vi "dfd_Create Rational Resampling Filter.vi"(6 "fs":dbl=1.0, 8 "error in (no error)":errorcluster, 10 "rational factor out":T6, 11 "validated numerator":dbl[](array[numeric])) -> (0 "error out":errorcluster, 3 "multirate filter out":T1={"mMRate_Structure"=enum."CIC", "mMRate_Mode"=0, "mMRate_Factor"=0, "mMRate_FIRParams"={"mMRate_FIR_H"=[], "mMRate_FIR_IsNyquist?"=FALSE, "mMRate_FIR_IsSymmetric?"=FALSE}, "mMRate_CICParams"={"mMRate_CIC_#Stage"=0, "mMRate_CIC_Lag"=0, "mMRate_CIC_Type"=enum."Lowpass"}, "mMRate_Order"=0, "mMRate_Version"="", "mMRate_Comments"="", "mMRate_RationalFactor"={"mMRate_L"=-1, "mMRate_M"=-1}, "mMRate_Fs"=0.0, "mMRate_Quantized?"=FALSE, "mMRate_QFilterGain"=1.0, "mMRate_CoefWl"=16, "mMRate_Scaling"={"mMRate_ScaleByPowerOf2?"=FALSE, "mMRate_ScaleType"=enum."Time Domain 1-Norm"}, "mMRate_InputWl"=0, "mMRate_OutputWl"=0, "mMRate_OutputMode"=enum."Nearest", "mMRate_MultMode"=enum."Full", "mMRate_BitPruning"=FALSE, "mMRate_GainWl"=16, "mMRate_OutputFwl"=0, "mMRate_SumIwl"=0, "mMRate_InputIwl "=16, "mMRate_SumWl"=32, "mMRate_CoefIwl"=0} {"mMRate_SumWl" min=1 max=32 step=1; "mMRate_InputIwl" min=1 max=32 step=1; "mMRate_GainWl" min=1 max=32 step=1; "mMRate_OutputWl" min=1 max=32 step=1; "mMRate_InputWl" min=1 max=32 step=1; "mMRate_CoefWl" min=1 max=32 step=1; "mMRate_Mode" items=["Default"=-1, "No Rate Change"=0, "Interpolation"=1, "Decimation"=2, "Interpolated"=3, "Rational"=4]})   [LabVIEW 2017, in "NI_DigFilterLicensed.lvlib"]
uses:
  <vilib>/addons/Digital Filter Design/NI_DigFilterLicensed.lvlib
  <vilib>/addons/Digital Filter Design/_Objects.llb/DFD Multirate Rational Factor.ctl
  <vilib>/addons/Digital Filter Design/_Objects.llb/DFD Multirate Filter Obj.ctl
  <vilib>/addons/Digital Filter Design/_Objects.llb/DFD Multirate Mode.ctl
  <vilib>/addons/Digital Filter Design/_Objects.llb/DFD Coef Norm Type.ctl
  <vilib>/addons/Digital Filter Design/_Objects.llb/DFD Round-off Mode.ctl
  <vilib>/addons/Digital Filter Design/_Objects.llb/DFD FXP MRate Multiply Mode.ctl
panel:
  in  "multirate filter":T1={"mMRate_Structure"=enum."IIR", "mMRate_Mode"=0, "mMRate_Factor"=-1, "mMRate_FIRParams"={"mMRate_FIR_H"=[], "mMRate_FIR_IsNyquist?"=FALSE, "mMRate_FIR_IsSymmetric?"=FALSE}, "mMRate_CICParams"={"mMRate_CIC_#Stage"=0, "mMRate_CIC_Lag"=0, "mMRate_CIC_Type"=enum."Lowpass"}, "mMRate_Order"=0, "mMRate_Version"="2.0", "mMRate_Comments"="", "mMRate_RationalFactor"={"mMRate_L"=-1, "mMRate_M"=-1}, "mMRate_Fs"=1.0, "mMRate_Quantized?"=FALSE, "mMRate_QFilterGain"=1.0, "mMRate_CoefWl"=16, "mMRate_Scaling"={"mMRate_ScaleByPowerOf2?"=FALSE, "mMRate_ScaleType"=enum."No Norm"}, "mMRate_InputWl"=16, "mMRate_OutputWl"=16, "mMRate_OutputMode"=enum."Truncation", "mMRate_MultMode"=enum."Truncated", "mMRate_BitPruning"=FALSE, "mMRate_GainWl"=16, "mMRate_OutputFwl"=0, "mMRate_SumIwl"=0, "mMRate_InputIwl "=16, "mMRate_SumWl"=32, "mMRate_CoefIwl"=0} {"mMRate_SumWl" min=1 max=32 step=1; "mMRate_InputIwl" min=1 max=32 step=1; "mMRate_GainWl" min=1 max=32 step=1; "mMRate_OutputWl" min=1 max=32 step=1; "mMRate_InputWl" min=1 max=32 step=1; "mMRate_CoefWl" min=1 max=32 step=1; "mMRate_Mode" items=["Default"=-1, "No Rate Change"=0, "Interpolation"=1, "Decimation"=2, "Interpolated"=3, "Rational"=4]}
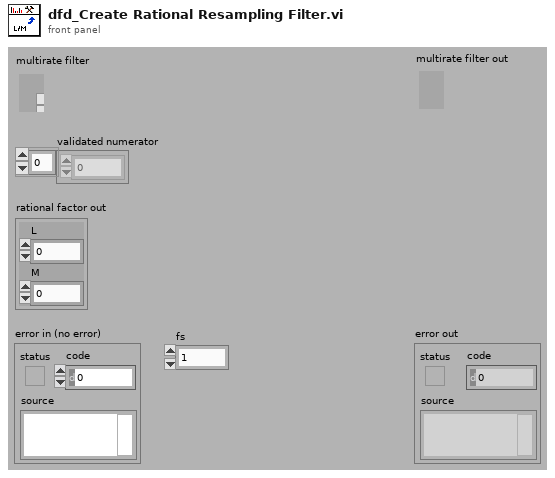
[diagram p1: front panel]
types:
  T1 = typedef "NI_DigFilterLicensed.lvlib/DFD Multirate Filter Obj.ctl" = cluster{"mMRate_Structure":enum16{"CIC", "FIR", "IIR", "Lattice"}, "mMRate_Mode":T2, "mMRate_Factor":i32, "mMRate_FIRParams":cluster{"mMRate_FIR_H":dbl[], "mMRate_FIR_IsNyquist?":bool, "mMRate_FIR_IsSymmetric?":bool}, "mMRate_CICParams":cluster{"mMRate_CIC_#Stage":i32, "mMRate_CIC_Lag":i32, "mMRate_CIC_Type":enum16{"Lowpass", "Highpass"}}, "mMRate_Order":i32, "mMRate_Version":string, "mMRate_Comments":string, "mMRate_RationalFactor":cluster{"mMRate_L":i32, "mMRate_M":i32}, "mMRate_Fs":dbl, "mMRate_Quantized?":bool, "mMRate_QFilterGain":dbl, "mMRate_CoefWl":i16, "mMRate_Scaling":cluster{"mMRate_ScaleByPowerOf2?":bool, "mMRate_ScaleType":T3}, "mMRate_InputWl":i16, "mMRate_OutputWl":i16, "mMRate_OutputMode":T4, "mMRate_MultMode":T5, "mMRate_BitPruning":bool, "mMRate_GainWl":i16, "mMRate_OutputFwl":i16, "mMRate_SumIwl":i16, "mMRate_InputIwl ":i16, "mMRate_SumWl":i16, "mMRate_CoefIwl":i16}
  T2 = typedef "NI_DigFilterLicensed.lvlib/DFD Multirate Mode.ctl" = i16
  T3 = typedef "NI_DigFilterLicensed.lvlib/DFD Coef Norm Type.ctl" = enum16{"No Norm", "Time Domain 1-Norm", "Time Domain 2-Norm", "Time Domain Inf-Norm"}
  T4 = typedef "NI_DigFilterLicensed.lvlib/DFD Round-off Mode.ctl" = enum16{"Nearest", "Truncation"}
  T5 = typedef "NI_DigFilterLicensed.lvlib/DFD FXP MRate Multiply Mode.ctl" = enum16{"Truncated", "Full"}
  T6 = typedef "NI_DigFilterLicensed.lvlib/DFD Multirate Rational Factor.ctl" = cluster{"L":i32, "M":i32}
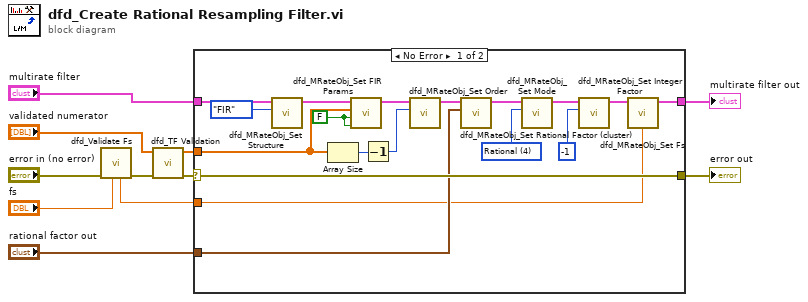
[diagram p0: block diagram]
diagram:
  n1 = call <vilib>:"dfd_Validate Fs.vi"("fs [Hz]"="fs", "error in (no error)"="error in (no error)") -> ("error out"=w2:errorcluster, "dup fs [Hz]"=w1:dbl)  [unwired: 8 in]
  n2 = call <vilib>:"dfd_TF Validation.vi"("error in (no error)"=w2, "numerator"="validated numerator") -> ("error out"=w7:errorcluster, "validated numerator"=w8:dbl[])  [unwired: 1 in, 4 out]
  n3 = case shown="No Error" w7 {
    selector: w7 -> [w28 w31]
    tunnel: "rational factor out" -> [w20 _]
    tunnel: [w13 w30] -> w10
    tunnel: w8 -> [w26 _]
    tunnel: [w28 w31] -> w6
    tunnel: "multirate filter" -> [w24 w30]
    tunnel: w1 -> [w12 _]
    frame No Error {
      w25 = T2 4 items=["Default"=-1, "No Rate Change"=0, "Interpolation"=1, "Decimation"=2, "Interpolated"=3, "Rational"=4] ("mode")
      w22 = FALSE ("is Nyquist?")
      n4 = call <vilib>:"dfd_MRateObj_Set Structure.vi"("structure"=enum16{"CIC", "FIR", "IIR", "Lattice"}."FIR", "multirate filter in"=w24) -> ("multirate filter out"=w23:T1)  [unwired: 9 out]
      n5 = Array Size(array=w26) -> (size(s)=w29:i32)
      n6 = call <vilib>:"dfd_MRateObj_Set FIR Params.vi"("is symmetric?"=w22, "is Nyquist?"=w22, "h(n)"=w26, "multirate filter in"=w23) -> ("multirate filter out"=w19:T1)  [unwired: 7 out]
      n7 = Decrement(x=w29) -> (x-1=w17:i32)
      n8 = call <vilib>:"dfd_MRateObj_Set Order.vi"("order"=w17, "multirate filter in"=w19) -> ("multirate filter out"=w18:T1)  [unwired: 9 out]
      n9 = call <vilib>:"dfd_MRateObj_Set Rational Factor (cluster).vi"("rational factor"=w20, "multirate filter in"=w18) -> ("multirate filter out"=w21:T1)  [unwired: 9 out]
      n10 = call <vilib>:"dfd_MRateObj_Set Mode.vi"("mode"=w25, "multirate filter in"=w21) -> ("multirate filter out"=w16:T1)  [unwired: 9 out]
      n11 = call <vilib>:"dfd_MRateObj_Set Integer Factor.vi"("factor"=-1, "multirate filter in"=w16) -> ("multirate filter out"=w14:T1)  [unwired: 9 out]
      n12 = call <vilib>:"dfd_MRateObj_Set Fs.vi"("fs"=w12, "multirate filter in"=w14) -> ("dup multirate filter"=w13:T1)  [unwired: 9 out]
    }
    frame Error {
    }
  }
  "multirate filter out" <- w10
  "error out" <- w6
